vi "ref_impedance_control_DOB_one motor_final_1.vi"() -> ()   [LabVIEW 2014]
uses:
  <vilib>/rvi/FXPMathLib/FxpSinAndCos/subVIs/nifxpmath_SinAndCos_SimConfig.ctl
  <vilib>/rvi/Emulation/niFpgaGetClockAttributes.vi
  <vilib>/rvi/Emulation/niFpgaSctlEmulationGetInTimedLoop.vi
  <vilib>/rvi/Emulation/niFpgaEmulationReportErrorSimple.vi
  <vilib>/rvi/eio/common/nirviEmuTemplateMethod_errors.vi
  <vilib>/rvi/Emulation/niFpgaProcessEmulError.vi
  <vilib>/rvi/Emulation/niFpgaCriticalErrorInLSC.vi
  <vilib>/rvi/interface/RandomDataEmulation/nirviRandomDataMultiElementFPGAFIFO.vi
  <instcachedir>/0/nirviRandomDataMultiElementFPGAFIFO_AD0CFC12EF974623A9C2E4184BC062B2.lvgen/nirviRandomDataMultiElementFPGAFIFO_AD0CFC12EF974623A9C2E4184BC062B2_010.vi
  <vilib>/rvi/interface/RandomDataEmulation/niFpgaRandomDataHandleErrors.vi
  <vilib>/rvi/FXPMathLib/FxpSinAndCos/simVIs/DllFxpSinAndCosTemp_sub.vi
  <vilib>/eio/EIONode/EIONode.xnode
  <vilib>/rvi/FXPMathLib/FxpMul/XNode/nifxpmath_Multiplier.xnode
  <vilib>/rvi/FXPMathLib/FxpSub/XNode/nifxpmath_Sub.xnode
  <vilib>/rvi/FXPMathLib/FxpAdd/XNode/nifxpmath_Add.xnode
  <vilib>/rvi/Analysis/measure/butterworth/XNode/niFpgaButterworthFilter.xnode
  <vilib>/rvi/DataTransferAndStorage/Container/XNode/niFpgaContainer.xnode
  <vilib>/rvi/interface/RandomDataEmulation/nirviRandomDataFpgaMultiElementTemplate.vi
  <vilib>/rvi/FXPMathLib/FxpSinAndCos/XNode/nifxpmath_SinAndCos.xnode
  <vilib>/rvi/FXPMathLib/sim/FxpSim.dll
panel:
  out "PID gain 1/2":bool
  in  "DOB set (5)":bool
  in  "DOB set (10)":bool
  in  "DOB set (40)":bool
  in  "DOB set (20)":bool
  in  "PID gain set 2":bool
  in  "PID gain set 1":bool
  in  "Chirp cmd/const freq":bool
  in  "x feedback (Encoder/Atom)":bool
  in  "D stroke lb (mm)":fxp<+/-,20,7>
  in  "Dar (mm)":fxp<+/-,20,7>
  out "fd":fxp<+/-,30,11>
  in  "Impedance/Force control":bool
  out "fd_imp ctrl":fxp<+/-,30,11>
  in  "Bv":fxp<+,20,5>
  in  "Kv":fxp<+,20,8>
  out "Da_d (mm/s)":fxp<+/-,21,9>
  out "Da (mm)":fxp<+/-,39,9>
  in  "x threshold (Counts)":i32
  out "D_ub":bool
  out "D_lb":bool
  in  "Q filter coe":i32[](array[numeric])=[-1066176100, 2139891176, 6687]
  in  "1st ord subsys coe":i32[](array[numeric])=[873670354, 100035735]
  out "DOB output":fxp<+/-,32,16>
  in  "Feedforward on/off":bool
  out "Q filter output":fxp<+/-,34,15>
  out "fr":fxp<+/-,30,11>
  out "Pn_inv*Q output":sgl format="%.2f"
  in  "K":sgl
  out "1st ord subsys output":fxp<+/-,36,20>
  out "2nd ord subsys output":sgl format="%.2f"
  in  "b1":sgl
  in  "b0":sgl
  in  "a0":sgl
  in  "a1":sgl
  in  "xi":fxp<+/-,20,10> format="%#_18g"
  in  "1/eta":fxp<+/-,20,4>=4.14569091796875 format="%#_18g"
  in  "ft_i clear":bool
  out "fr_d":fxp<+/-,38,22>
  in  "fd step size (N)":fxp<+/-,30,11>
  in  "fd (Step/Sin)":bool
  out "Avg M D_d (mm/s)":fxp<+/-,20,8>
  out "Avg M x_d (mm/s)":fxp<+/-,20,8>
  in  "Avg M_Ta (uSec)":u32=10
  in  "Velo est mthd (Avg M/T)":bool
  out "ft_d":fxp<+/-,20,13>
  out "f_d (N/s)":fxp<+/-,20,13>
  out "x_d (mm/s)":fxp<+/-,20,8>
  out "Atom Position":i32
  in  "Quad. Drv F_PID_d on/off":bool
  out "F_PID_d":fxp<+/-,32,22>
  in  "Load cell reset":bool
  in  "Load cell stop":bool
  in  "Load cell start":bool
  out "f_LC":fxp<+/-,31,16>
  in  "D stroke ub (mm)":fxp<+,19,6>
  in  "vq const (V)":fxp<+/-,20,6>
  in  "vd const (V)":fxp<+/-,20,6>
  in  "Quad. Drv./Const. vd,vq":bool
  out "D_d (mm/s)":fxp<+/-,20,8>
  in  "Sine amplitude (N)":fxp<+,20,10>
  in  "Sine freq (Hz)":sgl max=200
  out "Sine time (s)":fxp<+,47,13>
  in  "Atom Reset":bool
  out "x (mm)":fxp<+/-,36,8>
  in  "Coeffs Ini":bool
  in  "Encoder Reset":bool
  in  "Stop Motor":bool
  in  "Ki":fxp<+,15,7>
  in  "Kd":fxp<+,15,0>
  out "ft_i":fxp<+/-,30,12>
  in  "Kp":fxp<+,15,7>=0.375
  in  "k":fxp<+,20,6>
  out "f (N)":fxp<+/-,30,11>
  out "ft":fxp<+/-,30,11>
  out "F_PID":fxp<+/-,30,11>
  out "fd_force ctrl":fxp<+/-,30,11>
  out "Encoder Position":i32
  out "rad(NrTheta)":fxp<+/-,28,13> format="%.21g"
  out "D (mm)":fxp<+/-,38,8>
  out "omega (T method)":fxp<+/-,20,9>
  out "vq_F":fxp<+/-,20,6>
  out "vd_F":fxp<+/-,20,6>
  out "va":fxp<+/-,37,8>
  out "vb":fxp<+/-,38,9>
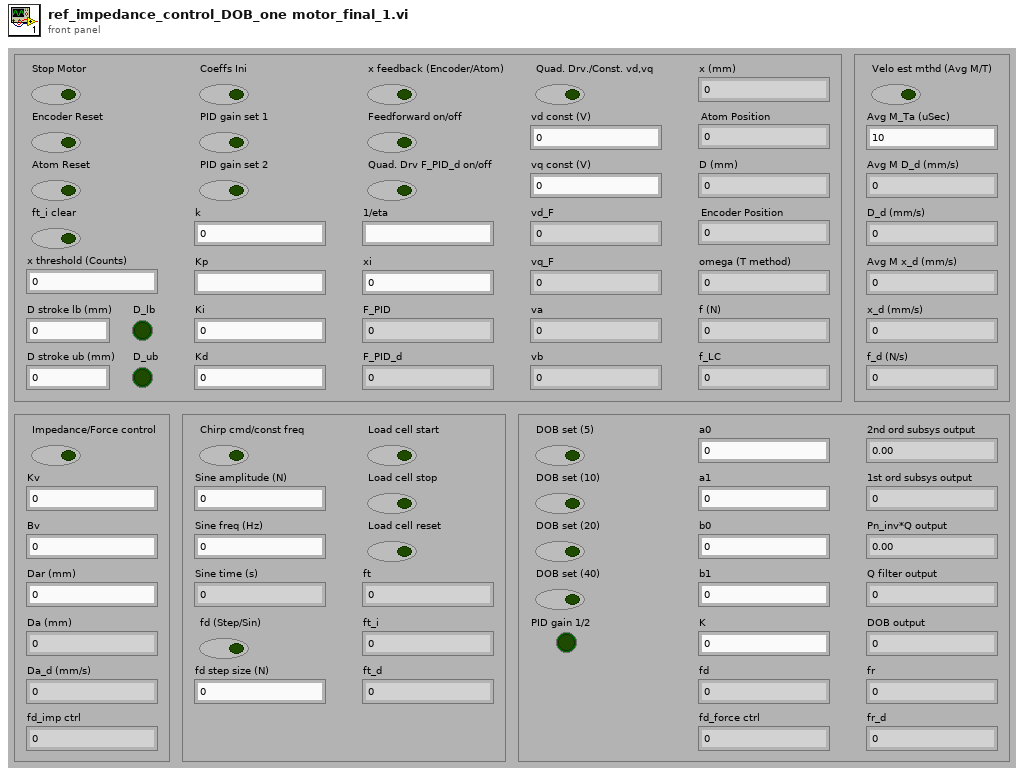
[diagram p1: front panel]
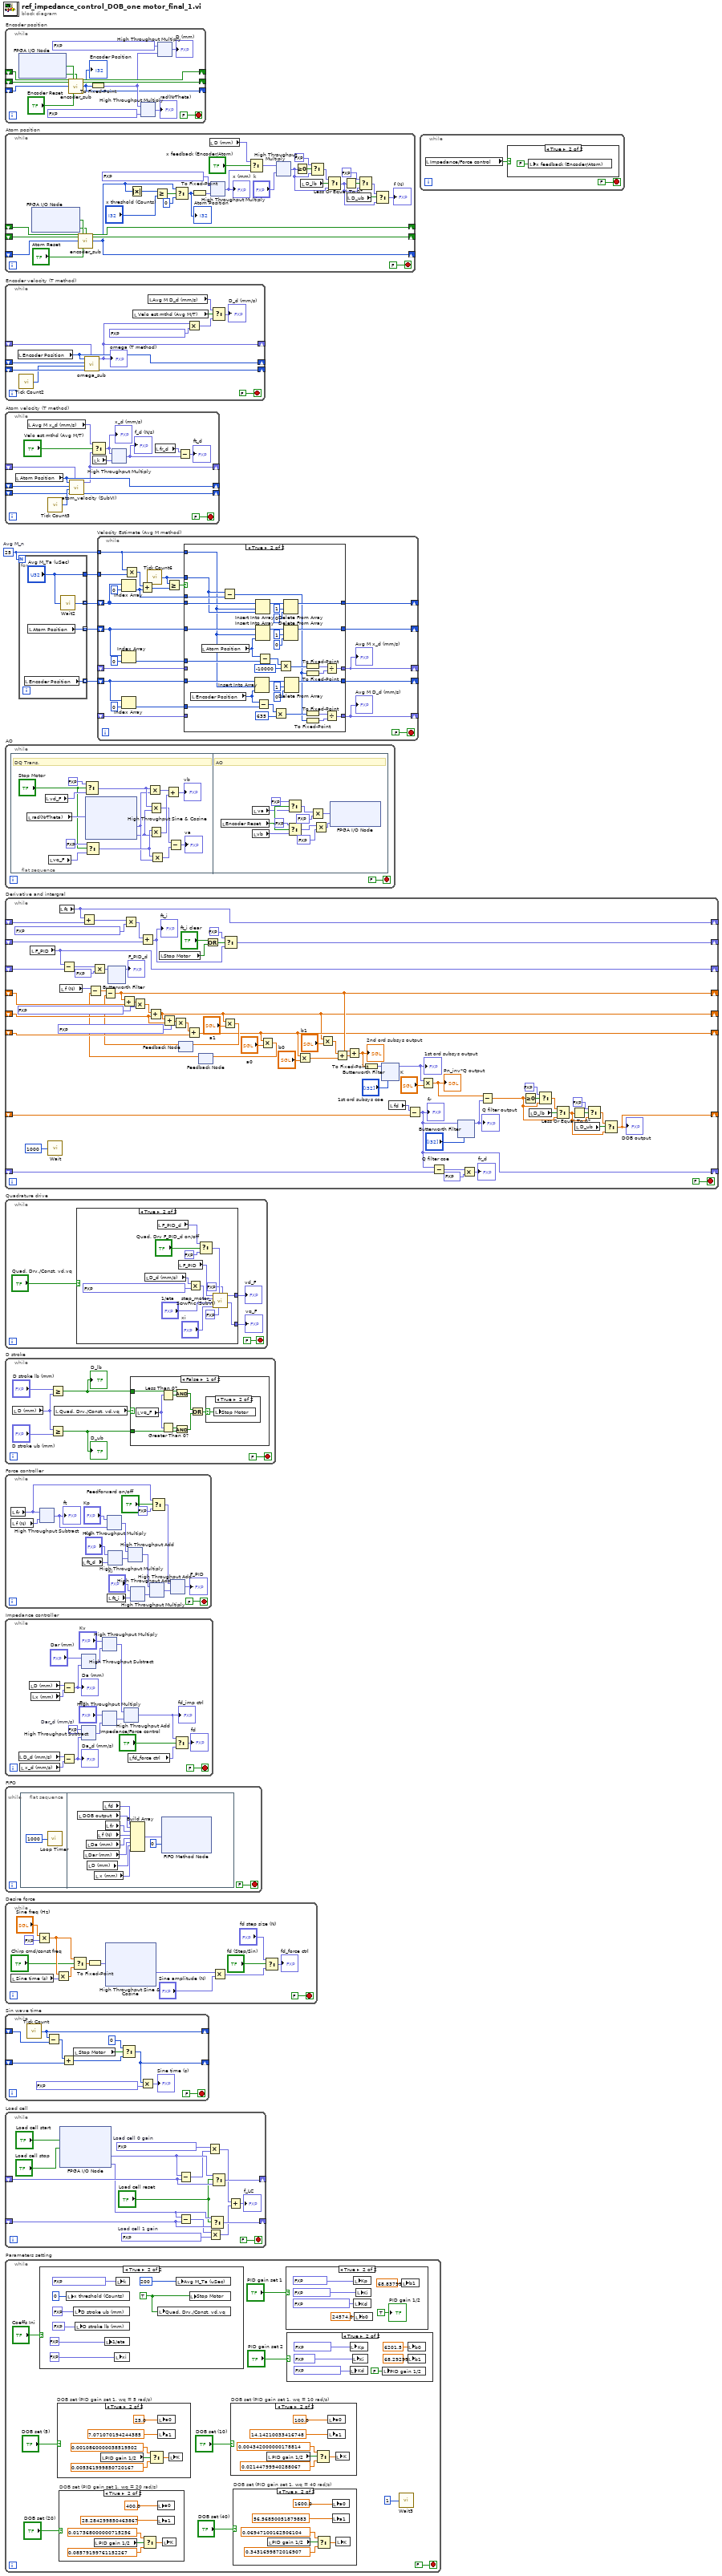
[diagram p0: block diagram]
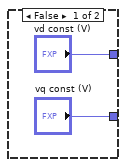
[diagram p13: hidden frame]
diagram:
  w3 = u32 25  # Avg M_n
  n1 = while "Encoder position" {
    shift-right: [w20] -> _
    shift-left: _ -> [w18]
    shift-right: [w19] -> _
    shift-left: _ -> [w17]
    shift-right: [w7] -> _
    shift-left: _ -> [w16]
    stop <- FALSE stop-if-true
    n2 = xnode "FPGA I/O Node"() -> ("Mod4/DI3"=w11:bool, "Mod4/DI4"=w10:bool)  [unwired: 2 in, 2 out]
    n3 = call "encoder_sub.vi"("A_pre"=w18, "B_pre"=w17, "Encoder Position_pre"=w16, "A input"=w11, "Encoder Position Reset"="Encoder Reset", "B input"=w10) -> ("A"=w20:bool, "B"=w19:bool, "Encoder Position (Counts)"=w7:i32)  [unwired: 19 in]
    "Encoder Position" <- w7
    n4 = To Fixed-Point(number=w7) -> (fixed-point=w8:fxp<+/-,18,18>)  [unwired: 1 in]
    n5 = xnode ("High Throughput Multiply")("x"=w8, "y"=fxp<+,20,-5> 0.025000005960464478) -> ("x*y"=→"rad(NrTheta)":fxp<+/-,28,13>)
    n6 = xnode ("High Throughput Multiply")("x"=fxp<+,20,-10> 0.0006349999457597733, "y"=w8) -> ("x*y"=→"D (mm)":fxp<+/-,38,8>)
  }
  n7 = while "Atom position" {
    shift-right: [w53] -> _
    shift-left: _ -> [w51]
    shift-right: [w52] -> _
    shift-left: _ -> [w50]
    shift-right: [w26] -> _
    shift-left: _ -> [w47]
    stop <- FALSE stop-if-true
    n8 = xnode "FPGA I/O Node"() -> ("Mod4/DI0"=w49:bool, "Mod4/DI1"=w48:bool)  [unwired: 2 in, 2 out]
    n9 = call "encoder_sub.vi"("A_pre"=w51, "B_pre"=w50, "Encoder Position_pre"=w47, "A input"=w49, "Encoder Position Reset"="Atom Reset", "B input"=w48) -> ("A"=w53:bool, "B"=w52:bool, "Encoder Position (Counts)"=w26:i32)  [unwired: 19 in]
    n10 = Absolute Value(x=w26) -> (abs(x)=w32:i32)
    n11 = Greater Or Equal?(x=w32, y="x threshold (Counts)") -> (x >= y?=w30:bool)
    n12 = Select(t=w26, s=w30, f=0) -> (s? t:f=w28:i32)
    "Atom Position" <- w28
    n13 = To Fixed-Point(number=w28) -> (fixed-point=w45:fxp<+/-,16,16>)  [unwired: 1 in]
    n14 = local read "D (mm)"() -> (w21:fxp<+/-,38,8>)
    n15 = xnode ("High Throughput Multiply")("x"=fxp<+/-,20,-8> -0.000999998301267624, "y"=w45) -> ("x*y"=w23:fxp<+/-,36,8>)
    "x (mm)" <- w23
    n16 = Select(t=w21, s="x feedback (Encoder/Atom)", f=w23) -> (s? t:f=w22:fxp<+/-,38,8>)
    n17 = xnode ("High Throughput Multiply")("x"=w22, "y"="k") -> ("x*y"=w33:fxp<+/-,30,11>)
    n18 = Greater Or Equal To 0?(x=w33) -> (x >= 0?=w44:bool)
    n19 = local read "D_lb"() -> (w43:bool)
    n20 = Select(t=fxp<+,1,1> 0.0, s=w44, f=w33) -> (s? t:f=w42:fxp<+/-,30,11>)
    n21 = Select(t=w42, s=w43, f=w33) -> (s? t:f=w36:fxp<+/-,30,11>)
    n22 = Less Or Equal To 0?(x=w36) -> (x <= 0?=w40:bool)
    n23 = local read "D_ub"() -> (w38:bool)
    n24 = Select(t=fxp<+,1,1> 0.0, s=w40, f=w36) -> (s? t:f=w37:fxp<+/-,30,11>)
    n25 = Select(t=w37, s=w38, f=w36) -> (s? t:f=→"f (N)":fxp<+/-,30,11>)
  }
  n26 = while "Encoder velocity (T method)" {
    shift-right: [w66] -> _
    shift-left: _ -> [w65]
    shift-right: [w64] -> _
    shift-left: _ -> [w63]
    shift-right: [w59] -> _
    shift-left: _ -> [w62]
    stop <- FALSE stop-if-true
    n27 = local read "Encoder Position"() -> (w66:i32)
    n28 = call "Tick Count2"() -> ("Tick Count(Ticks)"=w61:u32)
    n29 = call "omega_sub.vi"("omega_pre"=w62, "ticks_m_pre"=w63, "ticks"=w61, "count_pre"=w65, "count"=w66) -> ("ticks_m"=w64:u32, "omega"=w59:fxp<+/-,20,9>)  [unwired: 5 in]
    "omega (T method)" <- w59
    n30 = local read "Velo est mthd (Avg M/T)"() -> (w57:bool)
    n31 = local read "Avg M D_d (mm/s)"() -> (w56:fxp<+/-,20,8>)
    n32 = Multiply(x=w59, y=fxp<+,20,-1> 0.4042534828186035) -> (x*y=w55:fxp<+/-,20,8>)
    n33 = Select(t=w56, s=w57, f=w55) -> (s? t:f=→"D_d (mm/s)":fxp<+/-,20,8>)
  }
  n34 = while "Atom velocity (T method)" {
    shift-right: [w77] -> _
    shift-left: _ -> [w76]
    shift-right: [w73] -> _
    shift-left: _ -> [w74]
    shift-right: [w69] -> _
    shift-left: _ -> [w72]
    stop <- FALSE stop-if-true
    n35 = local read "Atom Position"() -> (w77:i32)
    n36 = local read "Avg M x_d (mm/s)"() -> (w71:fxp<+/-,20,8>)
    n37 = call "Tick Count3"() -> ("Tick Count(Ticks)"=w75:u32)
    n38 = call "atom_velocity (SubVI).vi"("omega_pre"=w72, "ticks_m_pre"=w74, "ticks"=w75, "count_pre"=w76, "count"=w77) -> ("ticks_m"=w73:u32, "omega"=w69:fxp<+/-,20,9>)  [unwired: 5 in]
    n39 = Select(t=w71, s="Velo est mthd (Avg M/T)", f=w69) -> (s? t:f=w67:fxp<+/-,21,9>)
    "x_d (mm/s)" <- w67
    n40 = local read "k"() -> (w81:fxp<+,20,6>)
    n41 = xnode ("High Throughput Multiply")("x"=w67, "y"=w81) -> ("x*y"=w79:fxp<+/-,20,13>)
    "f_d (N/s)" <- w79
    n42 = local read "fr_d"() -> (w80:fxp<+/-,38,22>)
    n43 = Subtract(x=w80, y=w79) -> (x-y=→"ft_d":fxp<+/-,20,13>)
  }
  n44 = while "AO" {
    stop <- FALSE stop-if-true
    n45 = flat-sequence {
      frame #0 {
        # "DQ Trans."
        n46 = local read "rad(NrTheta)"() -> (w98:fxp<+/-,28,13>)
        n47 = local read "vd_F"() -> (w97:fxp<+/-,20,6>)
        n48 = local read "vq_F"() -> (w95:fxp<+/-,20,6>)
        n49 = Select(t=fxp<+/-,14,0> 0.0, s="Stop Motor", f=w97) -> (s? t:f=w93:fxp<+/-,20,6>)
        n50 = xnode "High Throughput Sine & Cosine"("x (pi)"=w98) -> ("sin(x)"=w91:fxp<+/-,17,2>, "cos(x)"=w90:fxp<+/-,17,2>)
        n51 = Select(t=fxp<+/-,14,0> 0.0, s="Stop Motor", f=w95) -> (s? t:f=w92:fxp<+/-,20,6>)
        n52 = Multiply(x=w93, y=w91) -> (x*y=w89:fxp<+/-,37,8>)
        n53 = Multiply(x=w93, y=w90) -> (x*y=w87:fxp<+/-,37,8>)
        n54 = Multiply(x=w92, y=w90) -> (x*y=w88:fxp<+/-,37,8>)
        n55 = Multiply(x=w92, y=w91) -> (x*y=w86:fxp<+/-,37,8>)
        n56 = Add(x=w89, y=w88) -> (x+y=→"vb":fxp<+/-,38,9>)
        n57 = Subtract(x=w87, y=w86) -> (x-y=→"va":fxp<+/-,37,8>)
      }
      frame #1 {
        # "AO"
        n58 = local read "Encoder Reset"() -> (w134:bool)
        n59 = local read "vb"() -> (w132:fxp<+/-,38,9>)
        n60 = local read "va"() -> (w133:fxp<+/-,37,8>)
        n61 = Select(t=fxp<+,37,8> 5.0, s=w134, f=w133) -> (s? t:f=w136:fxp<+/-,38,9>)
        n62 = Select(t=fxp<+/-,38,9> 0.0, s=w134, f=w132) -> (s? t:f=w138:fxp<+/-,38,9>)
        n63 = Multiply(x=w136, y=fxp<+/-,20,1> -0.5) -> (x*y=w135:fxp<+/-,20,5>)
        n64 = Multiply(x=w138, y=fxp<+/-,20,1> -0.5) -> (x*y=w139:fxp<+/-,20,5>)
        n65 = xnode "FPGA I/O Node"("Mod8/AO4"=w135, "Mod8/AO5"=w139) -> ()  [unwired: 2 in, 2 out]
      }
    }
  }
  n66 = while "Derivative and intergral" {
    shift-right: [w197] -> _
    shift-left: _ -> [w196]
    shift-right: [w207] -> _
    shift-left: _ -> [w209]
    shift-right: [w201] -> _
    shift-left: _ -> [w202]
    shift-right: [w175] -> _
    shift-left: _ -> [w190]
    shift-right: [w172] -> _
    shift-left: _ -> [w186]
    shift-right: [w174] -> _
    shift-left: _ -> [w182]
    shift-right: [w144] -> _
    shift-left: _ -> [w162]
    shift-right: [w161] -> _
    shift-left: _ -> [w160]
    stop <- FALSE stop-if-true
    n67 = local read "F_PID"() -> (w201:fxp<+/-,30,11>)
    n68 = call "Wait"("Count(uSec)"=u32 1000 ("Count(mSec)")) -> ()  [unwired: 1 out]
    n69 = local read "ft"() -> (w197:fxp<+/-,30,11>)
    n70 = local read "f (N)"() -> (w192:fxp<+/-,30,11>)
    n71 = Subtract(x=w201, y=w202) -> (x-y=w205:fxp<+/-,31,12>)
    n72 = Add(x=w197, y=w196) -> (x+y=w199:fxp<+/-,31,12>)
    n73 = Multiply(x=w205, y=fxp<+,7,10> 1000.0) -> (x*y=w204:fxp<+/-,38,22>)
    n74 = xnode "Butterworth Filter"("input data"=w204) -> ("output data"=→"F_PID_d":fxp<+/-,32,22>)  [unwired: 2 in]
    n75 = Multiply(x=w199, y=fxp<+,20,-10> 0.0005000000819563866) -> (x*y=w200:fxp<+/-,20,2>)
    n76 = Add(x=w200, y=w209) -> (x+y=w208:fxp<+/-,30,12>)
    "ft_i" <- w208
    n77 = local read "Stop Motor"() -> (w143:bool)
    n78 = feedback #1() -> (w179:sgl)  [unwired: 1 in]
    n79 = feedback #2() -> (w176:sgl)  [unwired: 1 in]
    n80 = Subtract(x=w192, y=w176) -> (x-y=w191:sgl)
    n81 = Subtract(x=w191, y=w179) -> (x-y=w175:sgl)
    n82 = Add(x=w175, y=w190) -> (x+y=w189:sgl)
    n83 = Multiply(x=w189, y=fxp<+,20,-10> 0.0005000000819563866) -> (x*y=w187:sgl)
    n84 = Add(x=w187, y=w186) -> (x+y=w172:sgl)
    n85 = Add(x=w172, y=w186) -> (x+y=w185:sgl)
    n86 = Multiply(x=w185, y=fxp<+,20,-10> 0.0005000000819563866) -> (x*y=w183:sgl)
    n87 = Add(x=w183, y=w182) -> (x+y=w174:sgl)
    n88 = Or(x="ft_i clear", y=w143) -> (x .or. y?=w194:bool)
    n89 = Multiply(x=w172, y="a1") -> (x*y=w180:sgl)
    n90 = feedback-in #1(w180) -> ()
    n91 = Select(t=fxp<+,1,1> 0.0, s=w194, f=w208) -> (s? t:f=w207:fxp<+/-,30,12>)
    n92 = Multiply(x=w174, y="a0") -> (x*y=w177:sgl)
    n93 = feedback-in #2(w177) -> ()
    n94 = Multiply(x=w174, y="b0") -> (x*y=w169:sgl)
    n95 = Multiply(x=w172, y="b1") -> (x*y=w170:sgl)
    n96 = Add(x=w170, y=w169) -> (x+y=w168:sgl)
    n97 = Add(x=w175, y=w168) -> (x+y=w142:sgl)
    "2nd ord subsys output" <- w142
    n98 = To Fixed-Point(number=w142) -> (fixed-point=w141:fxp<+/-,32,16>)  [unwired: 1 in]
    n99 = xnode "Butterworth Filter"("input data"=w141, "scaled coefficients"="1st ord subsys coe") -> ("output data"=w167:fxp<+/-,36,20>)  [unwired: 1 in]
    "1st ord subsys output" <- w167
    n100 = local read "fd"() -> (w165:fxp<+/-,30,11>)
    n101 = Subtract(x=w165, y=w162) -> (x-y=w161:fxp<+/-,30,11>)
    "fr" <- w161
    n102 = Multiply(x=w167, y="K") -> (x*y=w164:sgl)
    "Pn_inv*Q output" <- w164
    n103 = Subtract(x=w161, y=w160) -> (x-y=w158:fxp<+/-,31,12>)
    n104 = xnode "Butterworth Filter"("input data"=w161, "scaled coefficients"="Q filter coe") -> ("output data"=w163:fxp<+/-,34,15>)  [unwired: 1 in]
    "Q filter output" <- w163
    n105 = Multiply(x=w158, y=fxp<+,7,10> 1000.0) -> (x*y=→"fr_d":fxp<+/-,38,22>)
    n106 = Subtract(x=w164, y=w163) -> (x-y=w147:sgl)
    n107 = Greater Or Equal To 0?(x=w147) -> (x >= 0?=w154:bool)
    n108 = local read "D_lb"() -> (w153:bool)
    n109 = Select(t=fxp<+,1,1> 0.0, s=w154, f=w147) -> (s? t:f=w152:sgl)
    n110 = Select(t=w152, s=w153, f=w147) -> (s? t:f=w148:sgl)
    n111 = Less Or Equal To 0?(x=w148) -> (x <= 0?=w151:bool)
    n112 = local read "D_ub"() -> (w150:bool)
    n113 = Select(t=fxp<+,1,1> 0.0, s=w151, f=w148) -> (s? t:f=w149:sgl)
    n114 = Select(t=w149, s=w150, f=w148) -> (s? t:f=w144:sgl)
    "DOB output" <- w144
  }
  n115 = while "Quadrature drive" {
    stop <- FALSE stop-if-true
    n116 = case shown="True" "Quad. Drv./Const. vd,vq" {
      tunnel: ["vd const (V)" w248] -> w236
      tunnel: ["vq const (V)" w247] -> w235
      frame False {
      }
      frame True {
        n117 = local read "D_d (mm/s)"() -> (w243:fxp<+/-,20,8>)
        n118 = local read "F_PID_d"() -> (w253:fxp<+/-,32,22>)
        n119 = local read "F_PID"() -> (w250:fxp<+/-,30,11>)
        n120 = Multiply(x=w243, y=fxp<+,20,-9> 0.0010000001639127731) -> (x*y=w242:fxp<+/-,40,-1>)
        n121 = Select(t=w253, s="Quad. Drv F_PID_d on/off", f=fxp<+,1,1> 0.0) -> (s? t:f=w251:fxp<+/-,32,22>)
        n122 = call "step_motor_ScrwFric (SubVI).vi"("D_dd"=fxp<+,1,1> 0.0, "F_Threshold"=fxp<+,1,1> 0.0, "F_d"=w251, "xi"="xi", "1/zeta"="1/eta", "D_d"=w242, "F"=w250) -> ("vq_F"=w247:fxp<+/-,20,6>, "vd_F"=w248:fxp<+/-,20,6>)  [unwired: 3 in]
      }
    }
    "vd_F" <- w236
    "vq_F" <- w235
  }
  n123 = while "D stroke" {
    stop <- FALSE stop-if-true
    n124 = local read "D (mm)"() -> (w255:fxp<+/-,38,8>)
    n125 = Greater Or Equal?(x="D stroke lb (mm)", y=w255) -> (x >= y?=w254:bool)
    "D_lb" <- w254
    n126 = Greater Or Equal?(x=w255, y="D stroke ub (mm)") -> (x >= y?=w257:bool)
    "D_ub" <- w257
    n127 = local read "Quad. Drv./Const. vd,vq"() -> (w260:bool)
    n128 = case shown="False" w260 {
      tunnel: w254 -> [w261 _]
      tunnel: w257 -> [w266 _]
      frame False {
        n129 = local read "vq_F"() -> (w267:fxp<+/-,20,6>)
        n130 = Less Than 0?(x=w267) -> (x < 0?=w262:bool)
        n131 = Greater Than 0?(x=w267) -> (x > 0?=w268:bool)
        n132 = And(x=w261, y=w262) -> (x .and. y?=w265:bool)
        n133 = And(x=w268, y=w266) -> (x .and. y?=w264:bool)
        n134 = Or(x=w265, y=w264) -> (x .or. y?=w263:bool)
        n135 = case shown="True" w263 {
          selector: w263 -> [_ w269]
          frame False {
          }
          frame True {
            n136 = local write "Stop Motor"(w269) -> ()
          }
        }
      }
      frame True {
      }
    }
  }
  n137 = while "Force controller" {
    stop <- FALSE stop-if-true
    n138 = local read "fr"() -> (w277:fxp<+/-,30,11>)
    n139 = local read "f (N)"() -> (w286:fxp<+/-,30,11>)
    n140 = xnode "High Throughput Subtract"("x"=w277, "y"=w286) -> ("x-y"=w273:fxp<+/-,30,11>)
    "ft" <- w273
    n141 = local read "ft_d"() -> (w278:fxp<+/-,20,13>)
    n142 = xnode ("High Throughput Multiply")("x"="Kp", "y"=w273) -> ("x*y"=w287:fxp<+/-,45,18>)
    n143 = local read "ft_i"() -> (w284:fxp<+/-,30,12>)
    n144 = xnode ("High Throughput Multiply")("x"="Kd", "y"=w278) -> ("x*y"=w282:fxp<+/-,35,13>)
    n145 = xnode ("High Throughput Add")("x"=w287, "y"=w282) -> ("x+y"=w285:fxp<+/-,46,19>)
    n146 = xnode ("High Throughput Multiply")("x"="Ki", "y"=w284) -> ("x*y"=w283:fxp<+/-,45,19>)
    n147 = xnode ("High Throughput Add")("x"=w285, "y"=w283) -> ("x+y"=w274:fxp<+/-,47,20>)
    n148 = Select(t=w277, s="Feedforward on/off", f=fxp<+,1,1> 0.0) -> (s? t:f=w276:fxp<+/-,30,11>)
    n149 = xnode ("High Throughput Add")("x"=w276, "y"=w274) -> ("x+y"=→"F_PID":fxp<+/-,30,11>)
  }
  n150 = while "Impedance controller" {
    stop <- FALSE stop-if-true
    w297 = fxp<+,1,1> 0.0  # Dar_d (mm/s)
    n151 = local read "D_d (mm/s)"() -> (w304:fxp<+/-,20,8>)
    n152 = local read "x_d (mm/s)"() -> (w303:fxp<+/-,20,8>)
    n153 = local read "D (mm)"() -> (w306:fxp<+/-,38,8>)
    n154 = local read "x (mm)"() -> (w305:fxp<+/-,36,8>)
    n155 = Subtract(x=w306, y=w305) -> (x-y=w301:fxp<+/-,39,9>)
    "Da (mm)" <- w301
    n156 = Subtract(x=w304, y=w303) -> (x-y=w298:fxp<+/-,21,9>)
    "Da_d (mm/s)" <- w298
    n157 = xnode "High Throughput Subtract"("x"="Dar (mm)", "y"=w301) -> ("x-y"=w299:fxp<+/-,40,10>)
    n158 = xnode "High Throughput Subtract"("x"=w297, "y"=w298) -> ("x-y"=w296:fxp<+/-,22,10>)
    n159 = xnode ("High Throughput Multiply")("x"="Kv", "y"=w299) -> ("x*y"=w294:fxp<+/-,60,18>)
    n160 = xnode ("High Throughput Multiply")("x"="Bv", "y"=w296) -> ("x*y"=w293:fxp<+/-,42,15>)
    n161 = xnode ("High Throughput Add")("x"=w294, "y"=w293) -> ("x+y"=w291:fxp<+/-,30,11>)
    "fd_imp ctrl" <- w291
    n162 = local read "fd_force ctrl"() -> (w290:fxp<+/-,30,11>)
    n163 = Select(t=w291, s="Impedance/Force control", f=w290) -> (s? t:f=→"fd":fxp<+/-,30,11>)
  }
  n164 = while "FIFO" {
    stop <- FALSE stop-if-true
    n165 = flat-sequence {
      frame #0 {
        n166 = call "Loop Timer"("Count(uSec)"=u32 1000 ("Loop Period (usec)")) -> ()  [unwired: 1 out]
      }
      frame #1 {
        n167 = local read "DOB output"() -> (w315:fxp<+/-,32,16>)
        n168 = local read "Dar (mm)"() -> (w309:fxp<+/-,20,7>)
        n169 = local read "Da (mm)"() -> (w310:fxp<+/-,39,9>)
        n170 = local read "D (mm)"() -> (w312:fxp<+/-,38,8>)
        n171 = local read "x (mm)"() -> (w311:fxp<+/-,36,8>)
        n172 = local read "f (N)"() -> (w313:fxp<+/-,30,11>)
        n173 = local read "fd"() -> (w316:fxp<+/-,30,11>)
        n174 = local read "fr"() -> (w314:fxp<+/-,30,11>)
        n175 = Build Array(w316, w315, w314, w313, w310, w309, w312, w311) -> (w317:fxp<+/-,46,16>[])
        n176 = xnode ("FIFO Method Node")("Element"=w317, "Timeout"=0) -> ()  [unwired: 1 in, 2 out]
      }
    }
  }
  n177 = while "Desire force" {
    stop <- FALSE stop-if-true
    n178 = local read "Sine time (s)"() -> (w332:fxp<+,47,13>)
    n179 = Multiply(x="Sine freq (Hz)", y=fxp<+,1,2> 2.0) -> (x*y=w323:sgl)
    n180 = Multiply(x=w323, y=w332) -> (x*y=w324:sgl)
    n181 = Select(t=w323, s="Chirp cmd/const freq", f=w324) -> (s? t:f=w321:sgl)
    n182 = To Fixed-Point(number=w321) -> (fixed-point=w320:fxp<+,64,22>)  [unwired: 1 in]
    n183 = xnode "High Throughput Sine & Cosine"("x (pi)"=w320) -> ("sin(x)"=w333:fxp<+/-,16,2>)  [unwired: 1 out]
    n184 = Multiply(x=w333, y="Sine amplitude (N)") -> (x*y=w328:fxp<+/-,30,11>)
    n185 = Select(t="fd step size (N)", s="fd (Step/Sin)", f=w328) -> (s? t:f=→"fd_force ctrl":fxp<+/-,30,11>)
  }
  n186 = while "Sin wave time" {
    shift-right: [w373] -> _
    shift-left: _ -> [w374]
    shift-right: [w365] -> _
    shift-left: _ -> [w370]
    stop <- FALSE stop-if-true
    n187 = call "Tick Count"() -> ("Tick Count(uSec)"=w373:u32)
    n188 = Subtract(x=w373, y=w374) -> (x-y=w371:u32)
    n189 = Add(x=w371, y=w370) -> (x+y=w369:u32)
    n190 = local read "Stop Motor"() -> (w368:bool)
    n191 = Select(t=u32 0, s=w368, f=w369) -> (s? t:f=w365:u32)
    n192 = Multiply(x=w365, y=fxp<+,15,-19> 1.00000761449337e-06) -> (x*y=→"Sine time (s)":fxp<+,47,13>)
  }
  n193 = while "Load cell" {
    shift-right: [w391] -> _
    shift-left: _ -> [w389]
    shift-right: [w388] -> _
    shift-left: _ -> [w386]
    stop <- FALSE stop-if-true
    w382 = fxp<+,36,18> 48771.92979812622  # Load cell 1 gain
    w383 = fxp<+,36,18> 47087.49039840698  # Load cell 0 gain
    n194 = xnode "FPGA I/O Node"("Mod6/Start"="Load cell start", "Mod6/Stop"="Load cell stop") -> ("Mod6/AI0"=w390:fxp<+/-,24,-4>, "Mod6/AI1"=w387:fxp<+/-,24,-4>)  [unwired: 4 in, 4 out]
    n195 = Subtract(x=w390, y=w389) -> (x-y=w385:fxp<+/-,25,-3>)
    n196 = Subtract(x=w387, y=w386) -> (x-y=w384:fxp<+/-,25,-3>)
    n197 = Multiply(x=w383, y=w385) -> (x*y=w381:fxp<+/-,30,15>)
    n198 = Multiply(x=w384, y=w382) -> (x*y=w380:fxp<+/-,30,15>)
    n199 = Select(t=w387, s="Load cell reset", f=w386) -> (s? t:f=w388:fxp<+/-,24,-4>)
    n200 = Select(t=w390, s="Load cell reset", f=w389) -> (s? t:f=w391:fxp<+/-,24,-4>)
    n201 = Add(x=w381, y=w380) -> (x+y=→"f_LC":fxp<+/-,31,16>)
  }
  n202 = while "Parameters setting" {
    stop <- FALSE stop-if-true
    n203 = case shown="True" "Coeffs Ini" {
      frame False {
      }
      frame True {
        w437 = TRUE ("Stop Motor_p")
        n204 = local write "x threshold (Counts)"(0 ("f_tolerance (N)")) -> ()
        n205 = local write "D stroke ub (mm)"(fxp<+,19,6> 10.0 ("Dp stroke")) -> ()
        n206 = local write "D stroke lb (mm)"(fxp<+/-,20,7> -10.0 ("Dp stroke")) -> ()
        n207 = local write "1/eta"(fxp<+/-,20,4> 1.0 ("fv")) -> ()
        n208 = local write "xi"(fxp<+/-,20,10> 0.0 ("xi")) -> ()
        n209 = local write "k"(fxp<+,20,6> 42.6290283203125 ("kp c")) -> ()
        n210 = local write "Quad. Drv./Const. vd,vq"(w437) -> ()
        n211 = local write "Avg M_Ta (uSec)"(u32 200 ("M_avg_Tc (uSec)")) -> ()
        n212 = local write "Stop Motor"(w437) -> ()
      }
    }
    n213 = case "DOB set (PID gain set 1, wq = 5 rad/s)" shown="True" "DOB set (5)" {
      frame False {
      }
      frame True {
        n214 = local read "PID gain 1/2"() -> (w401:bool)
        n215 = Select(t=sgl 0.001086 ("K/w1"), s=w401, f=sgl 0.005362 ("K/w1")) -> (s? t:f=w404:sgl)
        n216 = local write "a0"(sgl 25.0 ("a0")) -> ()
        n217 = local write "a1"(sgl 7.07107 ("a1")) -> ()
        n218 = local write "K"(w404) -> ()
      }
    }
    n219 = case "DOB set (PID gain set 1, wq = 20 rad/s)" shown="True" "DOB set (20)" {
      frame False {
      }
      frame True {
        n220 = local read "PID gain 1/2"() -> (w422:bool)
        n221 = Select(t=sgl 0.017368 ("K/w1"), s=w422, f=sgl 0.085792 ("K/w1")) -> (s? t:f=w419:sgl)
        n222 = local write "a0"(sgl 400.0 ("a0")) -> ()
        n223 = local write "a1"(sgl 28.2843 ("a1")) -> ()
        n224 = local write "K"(w419) -> ()
      }
    }
    n225 = case "DOB set (PID gain set 1, wq = 10 rad/s)" shown="True" "DOB set (10)" {
      frame False {
      }
      frame True {
        n226 = local read "PID gain 1/2"() -> (w410:bool)
        n227 = Select(t=sgl 0.004342 ("K/w1"), s=w410, f=sgl 0.021448 ("K/w1")) -> (s? t:f=w407:sgl)
        n228 = local write "a0"(sgl 100.0 ("a0")) -> ()
        n229 = local write "a1"(sgl 14.1421 ("a1")) -> ()
        n230 = local write "K"(w407) -> ()
      }
    }
    n231 = case "DOB set (PID gain set 1, wq = 40 rad/s)" shown="True" "DOB set (40)" {
      frame False {
      }
      frame True {
        n232 = local read "PID gain 1/2"() -> (w413:bool)
        n233 = Select(t=sgl 0.069471 ("K/w1"), s=w413, f=sgl 0.34317 ("K/w1")) -> (s? t:f=w416:sgl)
        n234 = local write "a0"(sgl 1600.0 ("a0")) -> ()
        n235 = local write "a1"(sgl 56.5685 ("a1")) -> ()
        n236 = local write "K"(w416) -> ()
      }
    }
    n237 = case shown="True" "PID gain set 1" {
      frame False {
      }
      frame True {
        n238 = local write "Kp"(fxp<+,15,7> 96.3046875 ("Kp")) -> ()
        n239 = local write "Kd"(fxp<+,15,0> 0.197052001953125 ("Kd")) -> ()
        n240 = local write "b0"(sgl 24574.0 ("b0")) -> ()
        n241 = local write "Ki"(fxp<+,15,7> 10.01953125 ("Ki")) -> ()
        n242 = local write "b1"(sgl 68.838 ("b1")) -> ()
        "PID gain 1/2" <- TRUE ("Boolean")
      }
    }
    n243 = case shown="True" "PID gain set 2" {
      frame False {
      }
      frame True {
        n244 = local write "Kp"(fxp<+,15,7> 19.75390625 ("Kp")) -> ()
        n245 = local write "Kd"(fxp<+,15,0> 0.198486328125 ("Kd")) -> ()
        n246 = local write "Ki"(fxp<+,15,7> 25.625 ("Ki")) -> ()
        n247 = local write "PID gain 1/2"(FALSE ("PID gain 1/2")) -> ()
        n248 = local write "b0"(sgl 6201.5 ("b0")) -> ()
        n249 = local write "b1"(sgl 68.293 ("b1")) -> ()
      }
    }
    n250 = call "Wait3"("Count(mSec)"=u8 1) -> ()  [unwired: 1 out]
  }
  n251 = for {
    N: w3 -> [_]
    tunnel: [w446] -> w5 mode=indexing
    tunnel: [w447] -> w4 mode=indexing
    tunnel: [w448] -> w2 mode=indexing
    tunnel: ["Avg M_Ta (uSec)"] -> w1
    n252 = local read "Encoder Position"() -> (w448:i32)
    n253 = local read "Atom Position"() -> (w447:i32)
    n254 = call "Wait2"("Count(uSec)"="Avg M_Ta (uSec)") -> ("Tick Count(uSec)"=w446:u32)
  }
  n255 = while "Velocity Estimate (Avg M method)" {
    tunnel: w3 -> [w466]
    shift-right: [w461] -> _
    shift-left: w5 -> [w465]
    shift-right: [w460] -> _
    shift-left: w4 -> [w464]
    shift-right: [w458] -> _
    shift-left: _ -> [w457]
    shift-right: [w455] -> _
    shift-left: w2 -> [w454]
    shift-right: [w452] -> _
    shift-left: _ -> [w451]
    tunnel: w1 -> [w450]
    stop <- FALSE stop-if-true
    n256 = Index Array(array=w465, index=0) -> (element=w462:u32)
    n257 = Index Array(array=w464, index=0) -> (element=w459:i32)
    n258 = Index Array(array=w454, index=0) -> (element=w453:i32)
    n259 = Multiply(x=w466, y=w450) -> (x*y=w471:u32)
    n260 = Add(x=w471, y=w462) -> (x+y=w468:u32)
    n261 = call "Tick Count6"() -> ("Tick Count(uSec)"=w463:u32)
    n262 = Greater Or Equal?(x=w463, y=w468) -> (x >= y?=w467:bool)
    n263 = case shown="True" w467 {
      tunnel: w466 -> [_ w484]
      tunnel: w465 -> [w476 w511]
      tunnel: w464 -> [w475 w510]
      tunnel: w463 -> [_ w499]
      tunnel: w462 -> [_ w500]
      tunnel: [w476 w503] -> w461
      tunnel: [w475 w502] -> w460
      tunnel: w459 -> [_ w497]
      tunnel: [w474 w495] -> w458
      tunnel: w457 -> [w474 _]
      tunnel: w454 -> [w473 w494]
      tunnel: [w473 w492] -> w455
      tunnel: w453 -> [_ w488]
      tunnel: [w472 w486] -> w452
      tunnel: w451 -> [w472 _]
      frame False {
      }
      frame True {
        n264 = local read "Encoder Position"() -> (w489:i32)
        n265 = local read "Atom Position"() -> (w498:i32)
        n266 = Subtract(x=w499, y=w500) -> (x-y=w478:u32)
        n267 = Insert Into Array(array=w494, index=w484, new element=w489) -> (w493:i32[])
        n268 = Insert Into Array(array=w511, index=w484, new element=w499) -> (w509:u32[])
        n269 = Insert Into Array(array=w510, index=w484, new element=w498) -> (w508:i32[])
        n270 = Subtract(x=w489, y=w488) -> (x-y=w487:i32)
        n271 = Subtract(x=w498, y=w497) -> (x-y=w496:i32)
        n272 = Multiply(x=w487, y=635) -> (x*y=w480:i32)
        n273 = Multiply(x=w496, y=-10000) -> (x*y=w483:i32)
        n274 = Delete From Array(array=w509, length=1, index=0) -> (array with subset deleted=w503:u32[])  [unwired: 1 out]
        n275 = Delete From Array(array=w508, length=1, index=0) -> (array with subset deleted=w502:i32[])  [unwired: 1 out]
        n276 = Delete From Array(array=w493, length=1, index=0) -> (array with subset deleted=w492:i32[])  [unwired: 1 out]
        n277 = To Fixed-Point(number=w483) -> (fixed-point=w482:fxp<+/-,32,32>)  [unwired: 1 in]
        n278 = To Fixed-Point(number=w478) -> (fixed-point=w481:fxp<+,32,32>)  [unwired: 1 in]
        n279 = To Fixed-Point(number=w480) -> (fixed-point=w479:fxp<+/-,32,32>)  [unwired: 1 in]
        n280 = To Fixed-Point(number=w478) -> (fixed-point=w477:fxp<+,32,32>)  [unwired: 1 in]
        n281 = Divide(x=w482, y=w481) -> (x/y=w495:fxp<+/-,20,8>)
        n282 = Divide(x=w479, y=w477) -> (x/y=w486:fxp<+/-,20,8>)
      }
    }
    "Avg M x_d (mm/s)" <- w458
    "Avg M D_d (mm/s)" <- w452
  }
  n283 = while {
    stop <- FALSE stop-if-true
    n284 = local read "Impedance/Force control"() -> (w513:bool)
    n285 = case shown="True" w513 {
      frame False {
      }
      frame True {
        n286 = local write "x feedback (Encoder/Atom)"(FALSE ("x feedback (Encoder/Atom)")) -> ()
      }
    }
  }
